vi "BIN_make_new_file.vi"(8 "error in":errorcluster, 9 "TAGs":string[](array[string]), 11 "FileName":path) -> (0 "error out":errorcluster, 3 "refnum out":refnum<file>)   [LabVIEW 2020, in "Sgraph_lib_V1.lvlib" / "DBAL-BIN.lvclass"]
doc: "Andre Koelewijn, 3 april 2021\n\nThis method is primary created for defragmentation purposes.\nIt creates a new BIN file and adds the TAGS header"
uses:
  DBAL-BIN.lvclass
  DBAL-BIN.lvclass/DBAL-BIN.ctl
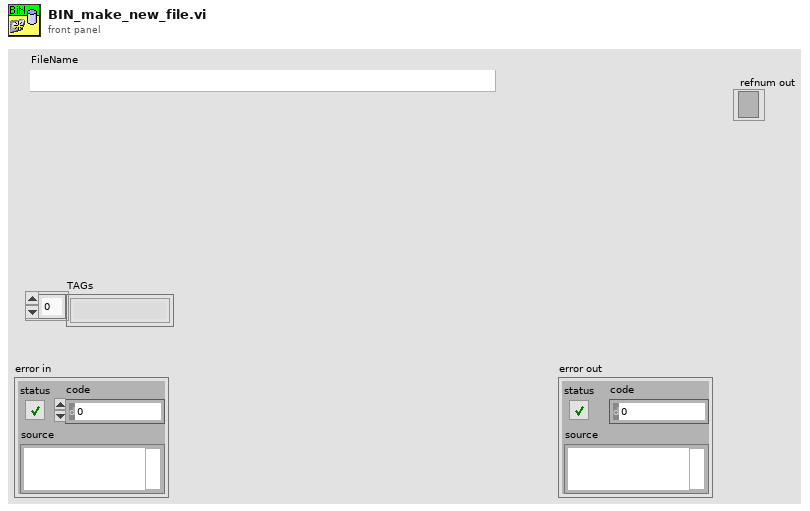
[diagram p1: front panel]
types:
  T1 = enum16{"open", "replace", "create", "open or create", "replace or create", "replace or create with confirmation"}
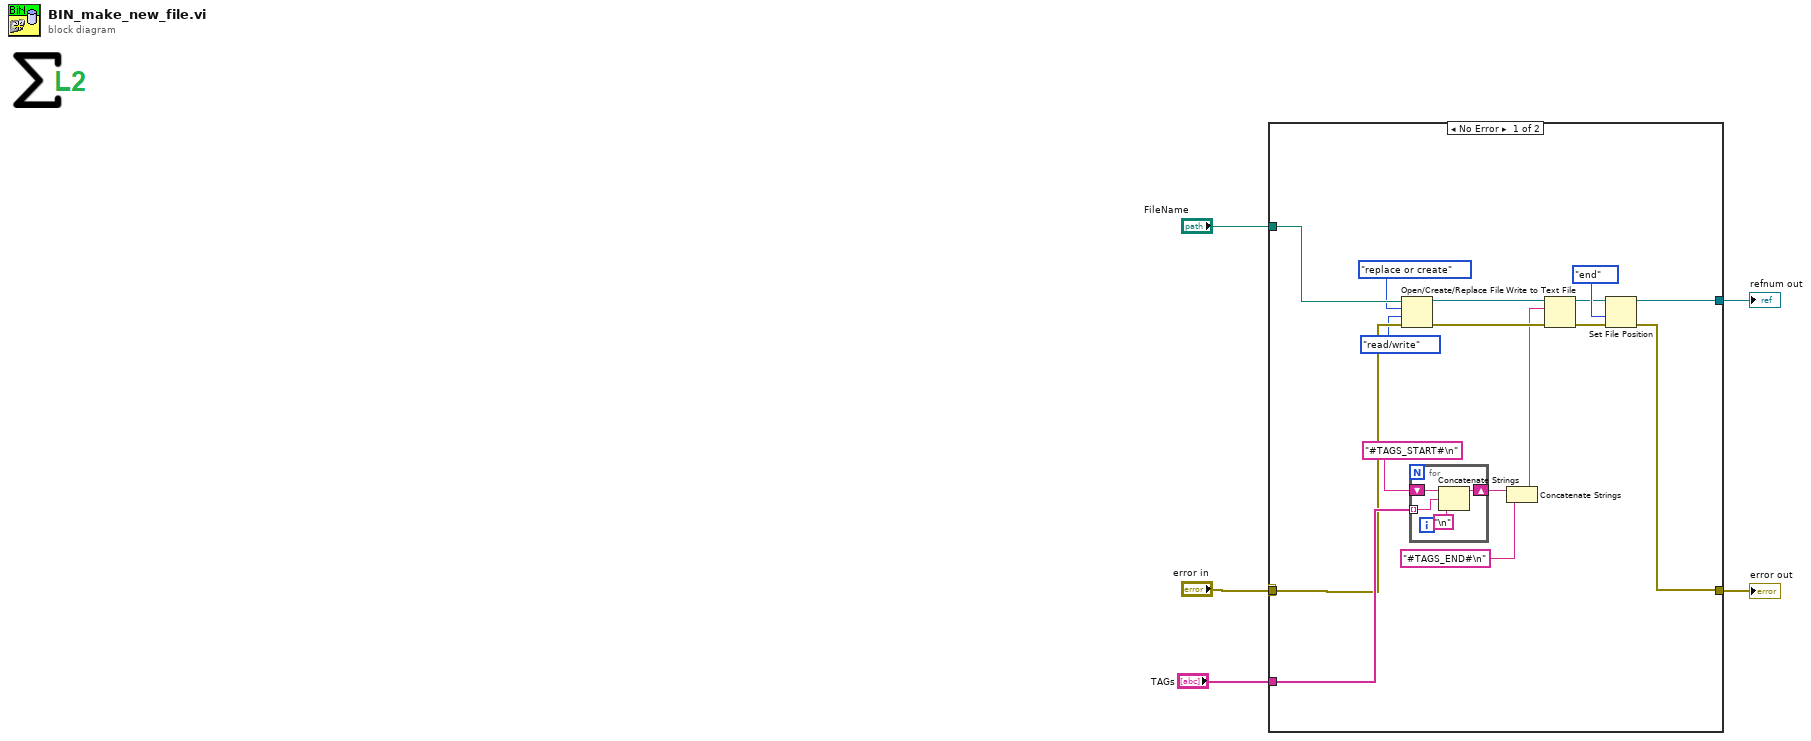
[diagram p0: block diagram]
diagram:
  n1 = case shown="No Error" "error in" {
    selector: "error in" -> [_ w26]
    tunnel: [w20 w26] -> w5
    tunnel: "FileName" -> [w17 _]
    tunnel: "TAGs" -> [w21 _]
    tunnel: [w19 _] -> w2
    tunnel: "error in" -> [w18 _]
    frame No Error {
      n2 = Open/Create/Replace File(file path (use dialog)=w17, error in=w18, operation (0:open)=T1."replace or create", access (0:read/write)=enum16{"read/write", "read-only", "write-only"}."read/write") -> (refnum out=w10:refnum<file>, error out=w8:errorcluster)  [unwired: 2 in, 1 out]
      n3 = for {
        tunnel: w21 -> [w24] mode=indexing
        shift-right: [w23] -> w13
        shift-left: "#TAGS_START#\n" -> [w25]
        n4 = Concatenate Strings(w25, w24, "\n") -> (w23:string)
      }
      n5 = Concatenate Strings(w13, "#TAGS_END#\n") -> (w7:string)
      n6 = Write to Text File(file (use dialog)=w10, text=w7, error in=w8) -> (refnum out=w6:refnum<file>, error out=w9:errorcluster)  [unwired: 1 in, 1 out]
      n7 = Set File Position(refnum=w6, from (0:start)=enum16{"start", "end", "current"}."end", error in=w9) -> (refnum out=w19:refnum<file>, error out=w20:errorcluster)  [unwired: 1 in]
    }
    frame Error {
    }
  }
  "error out" <- w5
  "refnum out" <- w2
